vi "Init Device.vi"(8 "error in (no error)":errorcluster, 11 "Device in":T1) -> (0 "error out":errorcluster, 3 "Device out":T1)   [LabVIEW 2015]
uses:
  typedefs/device.ctl
  <vilib>/Instr/_visa.llb/VISA Configure Serial Port (Instr).vi
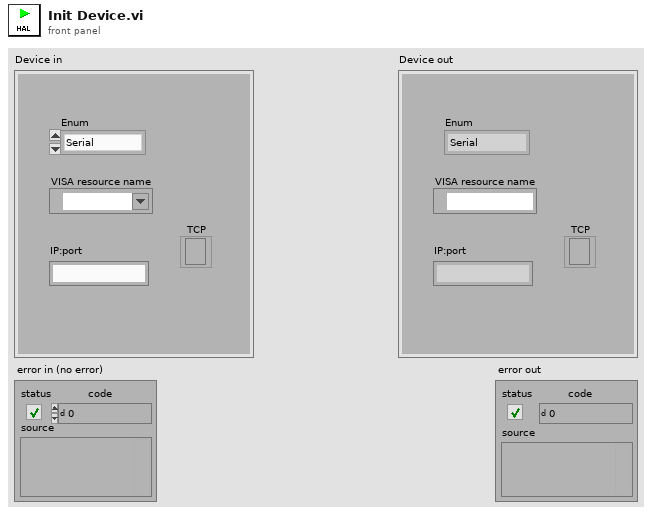
[diagram p1: front panel]
types:
  T1 = typedef "device.ctl" = cluster{"Enum":enum16{"Serial", "TCP/IP", "Mock"}, "IP:port":string, "VISA resource name":refnum<visa-resource-name>, "TCP":refnum<k5>}
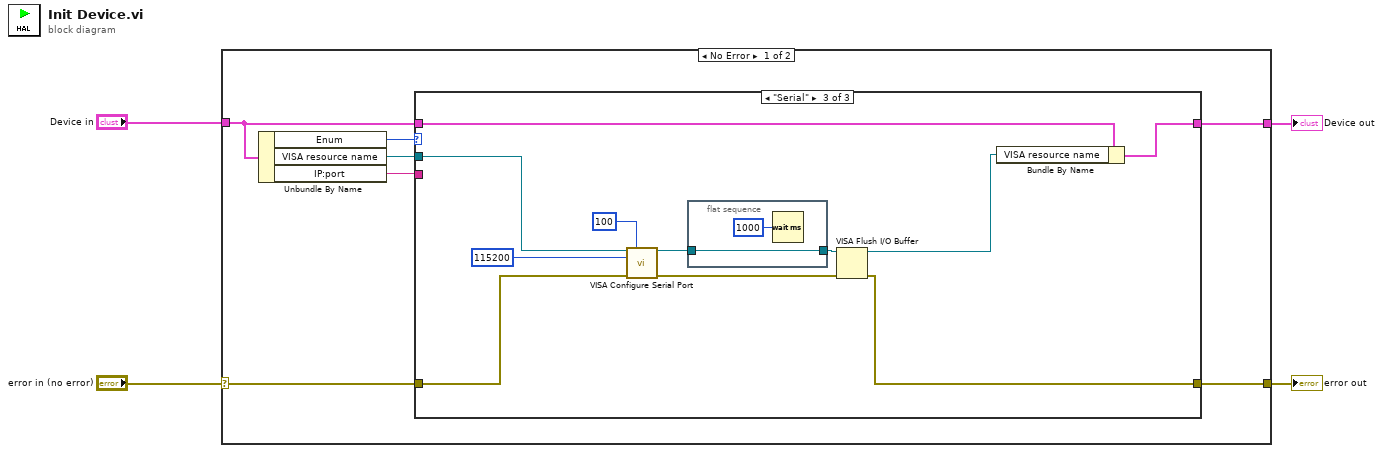
[diagram p0: block diagram]
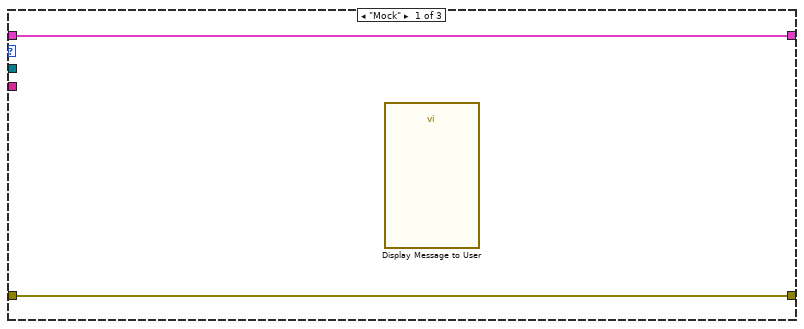
[diagram p2: hidden frame]
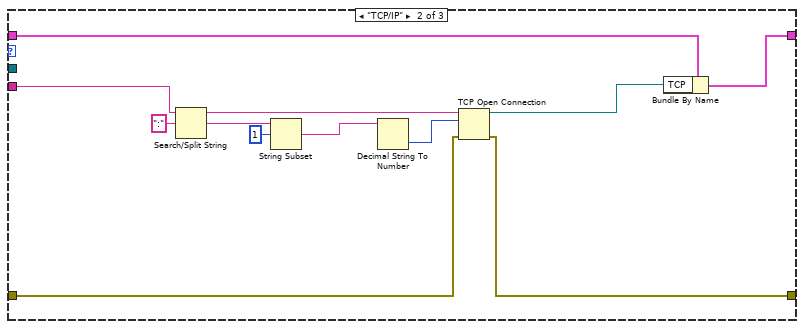
[diagram p3: hidden frame]
diagram:
  n1 = case shown="No Error" "error in (no error)" {
    selector: "error in (no error)" -> [w11 w39]
    tunnel: [w5 w40] -> w3
    tunnel: "Device in" -> [w6 w40]
    tunnel: [w10 w39] -> w1
    frame No Error {
      n2 = Unbundle By Name(w6) -> ("Enum"=w7:enum16{"Serial", "TCP/IP", "Mock"}, "VISA resource name"=w8:refnum<visa-resource-name>, "IP:port"=w9:string)
      n3 = case shown="\"Serial\"" w7 {
        tunnel: w9 -> [_ w20 _]
        tunnel: w8 -> [_ _ w29]
        tunnel: w11 -> [w13 w22 w31]
        tunnel: [w13 w21 w30] -> w10
        tunnel: w6 -> [w12 w15 w28]
        tunnel: [w12 w14 w27] -> w5
        frame "Mock" {
          n4 = call "Display Message to User"() -> ()  [unwired: 10 in, 2 out]
        }
        frame "TCP/IP" {
          n5 = Search/Split String(string=w20, search string/char (-)=":") -> (substring before match=w24:string, match + rest of string=w19:string)  [unwired: 1 in, 1 out]
          n6 = String Subset(string=w19, offset (0)=1) -> (substring=w17:string)  [unwired: 1 in]
          n7 = Decimal String To Number(string=w17) -> (number=w23:i32)  [unwired: 2 in, 1 out]
          n8 = TCP Open Connection(address=w24, remote port or service name=w23, error in (no error)=w22) -> (connection ID=w16:refnum<k5>, error out=w21:errorcluster)  [unwired: 2 in]
          n9 = Bundle By Name(cluster=w15, "TCP"=w16) -> (w14:T1)
        }
        frame "Serial" {
          n10 = call-poly "VISA Configure Serial Port"("VISA resource name"=w29, "timeout (10sec)"=u32 100, "baud rate (9600)"=u32 115200, "error in (no error)"=w31) -> ("VISA resource name out"=w33:refnum<visa-resource-name>, "error out"=w36:errorcluster)  [unwired: 5 in, 5 out]
          n11 = flat-sequence {
            tunnel: [w38] -> w34
            tunnel: w33 -> [w38]
            frame #0 {
              n12 = Wait (ms)(milliseconds to wait=u32 1000) -> ()  [unwired: 1 out]
            }
          }
          n13 = VISA Flush I/O Buffer(VISA resource name=w34, error in (no error)=w36) -> (VISA resource name out=w26:refnum<visa-resource-name>, error out=w30:errorcluster)  [unwired: 1 in]
          n14 = Bundle By Name(cluster=w28, "VISA resource name"=w26) -> (w27:T1)
        }
      }
    }
    frame Error {
    }
  }
  "error out" <- w1
  "Device out" <- w3
